vi "Simple Explorer.vi"(7 "Item Type":T1=enum."Setting", 8 "error in (no error)":errorcluster, 10 "Item ID":string, 11 "Configuration Session":refnum<class "Configuration Session.lvclass">) -> (0 "error out":errorcluster)   [LabVIEW 2017, in "DSF Simple Explorer.lvlib"]
uses:
  DSF Simple Explorer.lvlib
  Item Tree/ID to Tree Items/Tree Item Type.ctl
  VeriStand/Data Sharing Custom Device/Source/DSF Core.lvlibp/Classes/Configuration/Configuration Session.lvclass
  Main VI/Application Data.ctl
  Main VI/View Mode.ctl
  Item Tree/Create New Tree Item.vi
  VeriStand/Data Sharing Custom Device/Source/DSF Core.lvlibp/Classes/Configuration/Remove ID.vi
  VeriStand/Data Sharing Custom Device/Source/DSF Core.lvlibp/Classes/Configuration/Read Item.vi
  VeriStand/Data Sharing Custom Device/Source/DSF Core.lvlibp/Classes/Configuration/Read Plugin.vi
  VeriStand/Data Sharing Custom Device/Source/DSF Core.lvlibp/Classes/Configuration/Read Settings.vi
  VeriStand/Data Sharing Custom Device/Source/DSF Core.lvlibp/Classes/Configuration/Read Group.vi
  VeriStand/Data Sharing Custom Device/Source/DSF Core.lvlibp/Classes/Configuration/Read Transfer.vi
  VeriStand/Data Sharing Custom Device/Source/DSF Core.lvlibp/Classes/Configuration/Read Channel.vi
  Item Tree/Clear Tree.vi
  VeriStand/Data Sharing Custom Device/Source/DSF Core.lvlibp/Classes/Configuration/Read DSF Version.vi
  Value Tree/variant to tree resources/View Variant in Tree.vi
  VeriStand/Data Sharing Custom Device/Source/DSF Core.lvlibp/Classes/Configuration/Read Configuration Version.vi
  Item Tree/Get Item Type.vi
  Item Tree/Get Item Display Name.vi
  Item Tree/Get Parent.vi
  VeriStand/Data Sharing Custom Device/Source/DSF Core.lvlibp/Classes/Configuration/Append ID.vi
panel:
  in  "Item Tree":string(tree)
  in  "Value Tree":string(tree)
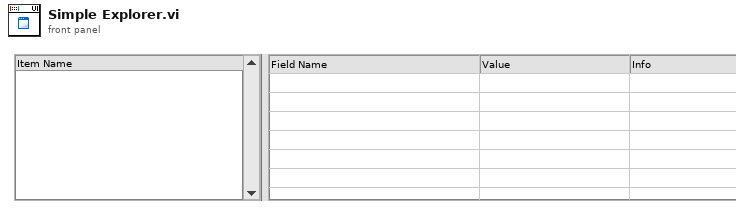
[diagram p1: front panel]
types:
  T1 = typedef "DSF Simple Explorer.lvlib/Tree Item Type.ctl" = enum16{"Plugin", "Group", "Transfer", "Channel", "Setting"}
  T2 = typedef "DSF Simple Explorer.lvlib/View Mode.ctl" = enum16{"Tree", "List"}
  T3 = typedef "DSF Simple Explorer.lvlib/Application Data.ctl" = cluster{"Item Tree Control":refnum<vi>, "Value Tree Control":refnum<vi>, "DSF Refnum":refnum<class "Configuration Session.lvclass">, "View State":T2}
  T4 = typedef "DSF Simple Explorer.lvlib/Tree Item.ctl" = cluster{"Left Cell String":string, "Child Text":string[], "Child Tag":string, "Glyph Index":i32}
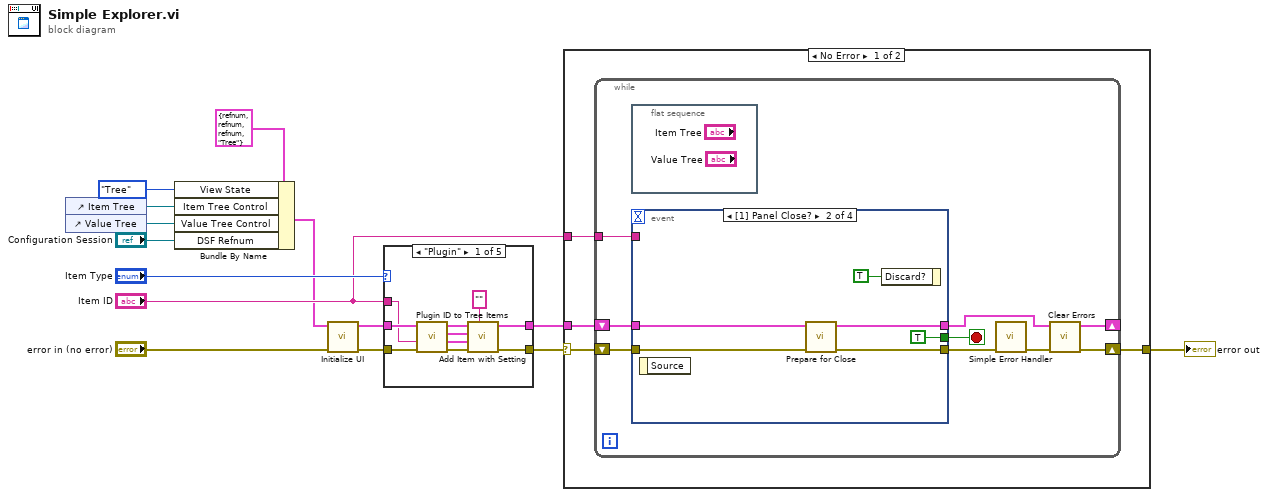
[diagram p0: block diagram]
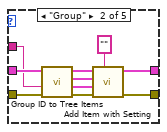
[diagram p2: hidden frame]
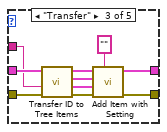
[diagram p3: hidden frame]
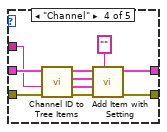
[diagram p4: hidden frame]
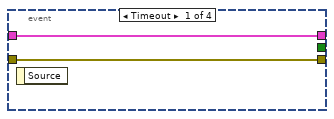
[diagram p6: hidden frame]
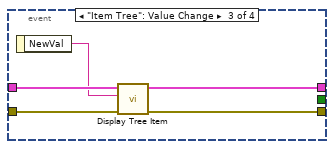
[diagram p7: hidden frame]
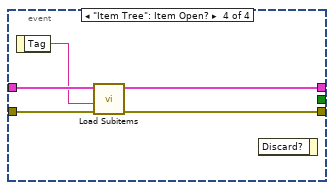
[diagram p8: hidden frame]
diagram:
  n1 = control-ref of="Item Tree"() -> (w13:refnum<vi>)
  n2 = control-ref of="Value Tree"() -> (w14:refnum<vi>)
  n3 = Bundle By Name(cluster=T3 {"Item Tree Control"=refnum, "Value Tree Control"=refnum, "DSF Refnum"=refnum, "View State"=enum."Tree"} ("Application Data in"), "View State"=View_Mode."Tree", "Item Tree Control"=w13, "Value Tree Control"=w14, "DSF Refnum"="Configuration Session") -> (w5:T3)
  n4 = call "Initialize UI.vi"("error in (no error)"="error in (no error)", "Application Data in"=w5) -> ("error out"=w10:errorcluster, "Application Data out"=w11:T3)  [unwired: 8 in]
  n5 = case shown="\"Plugin\"" "Item Type" {
    tunnel: w11 -> [w24 w30 w41 w48 w56]
    tunnel: w10 -> [w23 w31 w39 w49 w55]
    tunnel: [w18 w33 w43 w53 w55] -> w2
    tunnel: [w19 w34 w44 w54 w56] -> w9
    tunnel: "Item ID" -> [w22 w25 w38 w47 _]
    frame "Plugin" {
      n6 = call "Plugin ID to Tree Items.vi"("error in (no error)"=w23, "Plugin ID"=w22, "Application Data in"=w24) -> ("error out"=w20:errorcluster, "Settings"=w16:T4, "Item"=w17:T4, "Application Data out"=w21:T3)  [unwired: 5 in]
      n7 = call "Add Item with Setting.vi"("Parent Tag"="", "error in (no error)"=w20, "Setting"=w16, "Item"=w17, "Application Data in"=w21) -> ("error out"=w18:errorcluster, "Application Data out"=w19:T3)  [unwired: 4 in, 1 out]
    }
    frame "Group" {
      n8 = call "Group ID to Tree Items.vi"("error in (no error)"=w31, "Group ID"=w25, "Application Data in"=w30) -> ("error out"=w28:errorcluster, "Settings"=w26:T4, "Item"=w27:T4, "Application Data out"=w29:T3)  [unwired: 5 in]
      n9 = call "Add Item with Setting.vi"("Parent Tag"="", "error in (no error)"=w28, "Setting"=w26, "Item"=w27, "Application Data in"=w29) -> ("error out"=w33:errorcluster, "Application Data out"=w34:T3)  [unwired: 4 in, 1 out]
    }
    frame "Transfer" {
      n10 = call "Transfer ID to Tree Items.vi"("error in (no error)"=w39, "Transfer ID"=w38, "Application Data in"=w41) -> ("error out"=w37:errorcluster, "Settings"=w36:T4, "Item"=w35:T4, "Application Data out"=w40:T3)  [unwired: 5 in]
      n11 = call "Add Item with Setting.vi"("Parent Tag"="", "error in (no error)"=w37, "Setting"=w36, "Item"=w35, "Application Data in"=w40) -> ("error out"=w43:errorcluster, "Application Data out"=w44:T3)  [unwired: 4 in, 1 out]
    }
    frame "Channel" {
      n12 = call "Channel ID to Tree Items.vi"("error in (no error)"=w49, "Channel ID"=w47, "Application Data in"=w48) -> ("error out"=w50:errorcluster, "Settings"=w45:T4, "Item"=w46:T4, "Application Data out"=w51:T3)  [unwired: 5 in]
      n13 = call "Add Item with Setting.vi"("Parent Tag"="", "error in (no error)"=w50, "Setting"=w45, "Item"=w46, "Application Data in"=w51) -> ("error out"=w53:errorcluster, "Application Data out"=w54:T3)  [unwired: 4 in, 1 out]
    }
    frame "Setting" {
    }
  }
  n14 = case shown="No Error" w2 {
    selector: w2 -> [w57 w87]
    tunnel: [w60 w87] -> w1
    tunnel: w9 -> [w59 _]
    tunnel: "Item ID" -> [w58 _]
    frame No Error {
      n15 = while {
        shift-right: [w62] -> w60
        shift-left: w57 -> [w67]
        shift-right: [w63] -> _
        shift-left: w59 -> [w64]
        tunnel: w58 -> [w61]
        stop <- w68 stop-if-true
        n16 = flat-sequence {
          frame #0 {
          }
        }
        n17 = event shown="[1] Panel Close?" {
          selector: _ -> [_ _ _ _]
          dyn-events: _ -> [_ _ _ _]
          timeout: _ -> [_ _ _ _]
          tunnel: [_ TRUE _ _] -> w68
          tunnel: w67 -> [w70 w75 w81 w86]
          tunnel: [w70 w72 w80 w85] -> w65
          tunnel: w64 -> [w69 w73 w78 w84]
          tunnel: [w69 w71 w79 w83] -> w63
          tunnel: w61 -> [_ _ _ _]
          event Timeout {
            n18 = event-data() -> ()  [unwired: 1 in, 1 out]
          }
          event Panel Close? {
            n19 = event-data() -> ()  [unwired: 1 in, 1 out]
            n20 = call "Prepare for Close.vi"("error in (no error)"=w75, "Application Data in"=w73) -> ("error out"=w72:errorcluster, "Application Data out"=w71:T3)  [unwired: 8 in]
            n21 = event-data("Discard?"=TRUE) -> ()  [unwired: 1 in, 1 out]
          }
          event "Item Tree": Value Change {
            n22 = event-data() -> ("NewVal"=w77:string)  [unwired: 1 in]
            n23 = call "Display Tree Item.vi"("error in (no error)"=w81, "Tag"=w77, "Application Data in"=w78) -> ("error out"=w80:errorcluster, "Application Data out"=w79:T3)  [unwired: 7 in]
          }
          event "Item Tree": Item Open? {
            n24 = event-data() -> ("Tag"=w82:string)  [unwired: 1 in]
            n25 = call "Load Subitems.vi"("error in (no error)"=w86, "Tag"=w82, "Application Data in"=w84) -> ("error out"=w85:errorcluster, "Application Data out"=w83:T3)  [unwired: 6 in, 1 out]
            n26 = event-data() -> ()  [unwired: 2 in, 1 out]
          }
        }
        n27 = call <vilib>:"Simple Error Handler.vi"("error in (no error)"=w65) -> ("error out"=w66:errorcluster)  [unwired: 4 in, 4 out]
        n28 = call <vilib>:"Clear Errors.vi"("error in (no error)"=w66) -> ("error out"=w62:errorcluster)  [unwired: 5 in, 1 out]
      }
    }
    frame Error {
    }
  }
  "error out" <- w1
